vi "Save Image.vi"(8 "error in (no error)":errorcluster, 9 "Save Path":path, 10 "Image":T1, 11 "Camera Driver in":refnum<class "Camera Driver.lvclass">) -> (0 "error out":errorcluster, 3 "Camera Driver out":refnum<class "Camera Driver.lvclass">)   [LabVIEW 2022 SP3, in "Camera Driver.lvclass"]
uses:
  Camera Driver.lvclass
  <vilib>/vision/Image Controls.llb/IMAQ Image.ctl
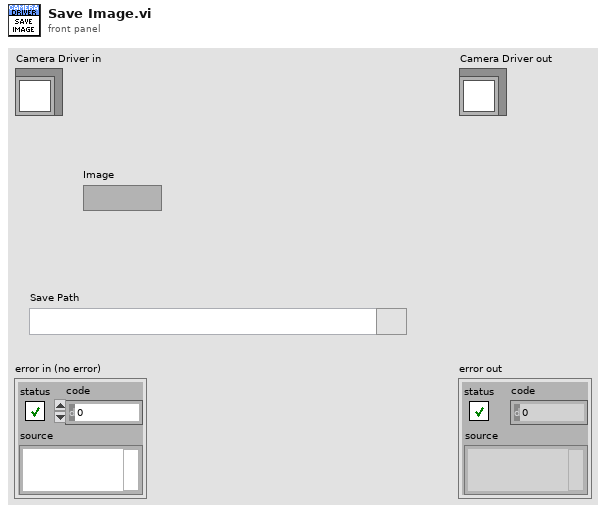
[diagram p1: front panel]
types:
  T1 = typedef "IMAQ Image.ctl" = refnum<image>
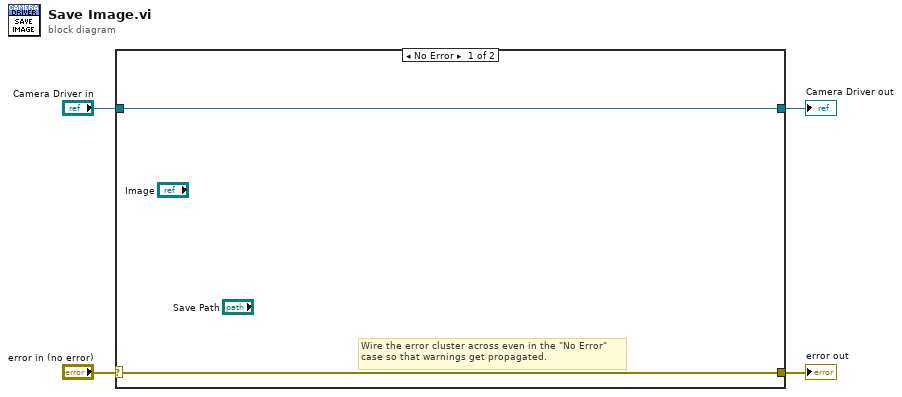
[diagram p0: block diagram]
diagram:
  n1 = case shown="No Error" "error in (no error)" {
    selector: "error in (no error)" -> [w5 w8]
    tunnel: [w5 w8] -> w3
    tunnel: [w6 w7] -> w1
    tunnel: "Camera Driver in" -> [w6 w7]
    frame No Error {
      # "Wire the error cluster across even in the \"No Error\"\ncase so that warnings get propagated."
    }
    frame Error {
    }
  }
  "error out" <- w3
  "Camera Driver out" <- w1
